vi "Lockin.DAQ.Get Calibration.vi"(8 "error in (no error)":errorcluster, 11 "Lockin.DAQ in":refnum<class "Instrument.DAQ.lvclass">) -> (0 "error out":errorcluster, 2 "Cal Info":T1[](array[typedef]) {"SelfCal.LastDate/Time" format="%<%I:%M %p\n%m/%d/%Y>T"}, 3 "Lockin.DAQ out":refnum<class "Instrument.DAQ.lvclass">)   [LabVIEW 2019, in "Instrument.DAQ.lvclass"]
uses:
  Instrument.DAQ.lvclass
  Typedefs/Cal Info - Cluster.ctl
  Instrument.DAQ.lvclass/Instrument.DAQ.ctl
  <resource>/objmgr/daqmx.rc
  <userlib>/_OpenG.lib/array/array.llb/Remove Duplicates from 1D Array (String)__ogtk.vi
panel:
  out "cal due?":bool
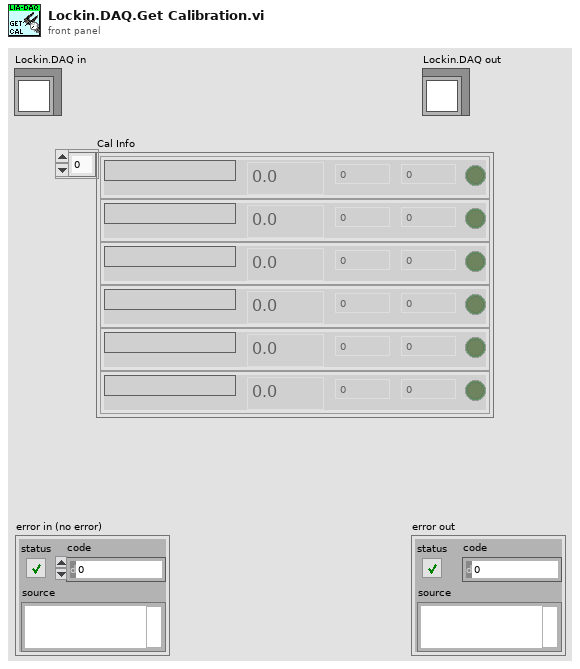
[diagram p1: front panel]
types:
  T1 = typedef "Instrument.DAQ.lvclass/Cal Info - Cluster.ctl" = cluster{"Active Device":string, "SelfCal.LastDate/Time":dbl, "SelfCal.LastTemp":dbl, "DevTemp":dbl, "calibration due?":bool}
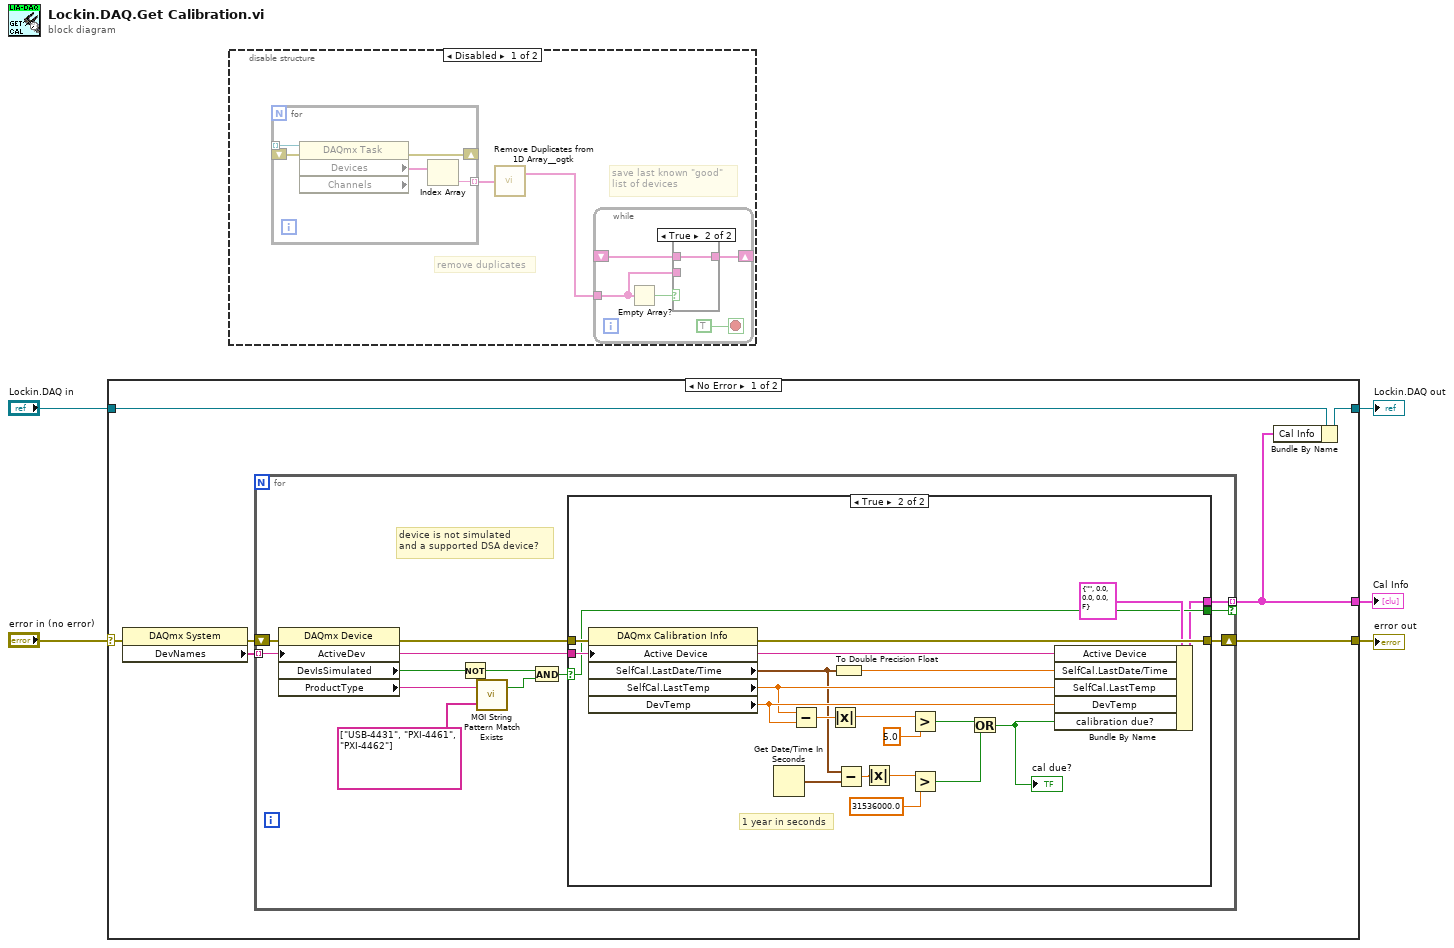
[diagram p0: block diagram]
diagram:
  n1 = case shown="No Error" "error in (no error)" {
    selector: "error in (no error)" -> [w7 w47]
    tunnel: [w12 w47] -> w5
    tunnel: "Lockin.DAQ in" -> [w11 w48]
    tunnel: [w10 w48] -> w3
    tunnel: [w6 _] -> w2
    frame No Error {
      n2 = property class="DAQmx System"(error in=w7) -> (error out=w8:errorcluster, "DevNames"=w9:tag[])  [unwired: 1 in, 1 out]
      n3 = for {
        tunnel: [w23] -> w6 mode=indexing if=w13
        shift-right: [w24] -> w12
        shift-left: w8 -> [w22]
        tunnel: w9 -> [w21] mode=indexing
        # "device is not simulated\nand a supported DSA device?"
        n4 = property class="DAQmx Device"(error in=w22, "ActiveDev"=w21) -> (error out=w20:errorcluster, "DevIsSimulated"=w19:bool, "ProductType"=w15:string)  [unwired: 1 in, 1 out]
        n5 = Not(x=w19) -> (.not. x?=w17:bool)
        n6 = call <userlib>:"MGI String Pattern Match Exists.vi"("Patterns to Try"=string[] ["USB-4431", "PXI-4461", "PXI-4462"], "String"=w15) -> ("Match Found"=w14:bool)  [unwired: 1 out]
        n7 = And(x=w17, y=w14) -> (x .and. y?=w18:bool)
        n8 = case shown="True" w18 {
          selector: w18 -> [w25 w28]
          tunnel: [w26 w46] -> w24
          tunnel: [_ w27] -> w23
          tunnel: w21 -> [_ w30]
          tunnel: w20 -> [w26 w29]
          tunnel: [w25 w28] -> w13
          frame False {
          }
          frame True {
            # "1 year in seconds"
            n9 = property class="DAQmx Calibration Info"(error in=w29, "Active Device"=w30) -> (error out=w46:errorcluster, "SelfCal.LastDate/Time"=w38:timestamp, "SelfCal.LastTemp"=w39:dbl, "DevTemp"=w40:dbl)  [unwired: 1 in, 1 out]
            n10 = Get Date/Time In Seconds() -> (seconds since 1Jan1904=w37:timestamp)
            n11 = Subtract(x=w39, y=w40) -> (x-y=w45:dbl)
            n12 = Absolute Value(x=w45) -> (abs(x)=w44:dbl)
            n13 = To Double Precision Float(number=w38) -> (double precision float=w41:dbl)
            n14 = Subtract(x=w38, y=w37) -> (x-y=w36:dbl)
            n15 = Absolute Value(x=w36) -> (abs(x)=w35:dbl)
            n16 = Greater?(x=w44, y=5.0) -> (0:w34:bool)
            n17 = Greater?(x=w35, y=31536000.0) -> (0:w33:bool)
            n18 = Or(x=w34, y=w33) -> (x .or. y?=w32:bool)
            "cal due?" <- w32
            n19 = Bundle By Name(cluster=T1 {"Active Device"="", "SelfCal.LastDate/Time"=0.0, "SelfCal.LastTemp"=0.0, "DevTemp"=0.0, "calibration due?"=FALSE} ("Calibration"), "Active Device"=w30, "SelfCal.LastDate/Time"=w41, "SelfCal.LastTemp"=w39, "DevTemp"=w40, "calibration due?"=w32) -> (w27:T1)
          }
        }
      }
      n20 = Bundle By Name(cluster=w11, "Cal Info"=w6) -> (w10:refnum<class "Instrument.DAQ.lvclass">)
    }
    frame Error {
    }
  }
  "error out" <- w5
  "Cal Info" <- w2
  "Lockin.DAQ out" <- w3
  n21 = disable-structure shown="Disabled" {
    frame Disabled {
      # "save last known \"good\"\nlist of devices"
      # "remove duplicates"
      n22 = for {
        tunnel: [w53] -> w50 mode=indexing
        shift-right: [w54] -> _
        shift-left: _ -> [w55]
        tunnel: _ -> [w51] mode=indexing
        n23 = property class="DAQmx Task" props=["Devices", "Channels"](reference=w51, error in=w55) -> (error out=w54:errorcluster, "Devices"=w52:tag[])  [unwired: 2 out]
        n24 = Index Array(array=w52) -> (element=w53:tag)  [unwired: 1 in]
      }
      n25 = call-poly <userlib>:"Remove Duplicates from 1D Array__ogtk.vi"("Input Array"=w50) -> ("Output Array"=w49:string[])  [unwired: 1 out]
      n26 = while {
        shift-right: [w58] -> _
        shift-left: _ -> [w56]
        tunnel: w49 -> [w57]
        stop <- TRUE stop-if-true
        n27 = Empty Array?(array=w57) -> (empty?=w59:bool)
        n28 = case shown="True" w59 {
          tunnel: [w61 w62] -> w58
          tunnel: w57 -> [w61 _]
          tunnel: w56 -> [_ w62]
          frame False {
          }
          frame True {
          }
        }
      }
    }
    frame Enabled {
    }
  }
